vi "Sub Initialize.vi"(6 "Controller name":string, 8 "error in (no error)":errorcluster, 11 "Instrument Recorder in":refnum<class "DataSocket Client.lvclass">) -> (0 "error out":errorcluster, 2 "Initialize Result":refnum<class "Acquired Result.lvclass">, 3 "Instrument Recorder out":refnum<class "DataSocket Client.lvclass">)   [LabVIEW 2021, in "DataSocket Client.lvclass"]
uses:
  DataSocket Client.lvclass
  DataSocket Client.lvclass/DataSocket Client.ctl
  NHMFL_Core/Libraries/Instruments/Results/Start Stream Result/Start Stream Result.lvclass
  C:/GitHub/NHMFL_Core/Libraries/Instruments/Results/Acquired Result/Acquired Result.lvclass
  C:/GitHub/LabActor/Publish-Subscribe/Interfaces/Information/Information.lvclass
  C:/GitHub/NHMFL_Core/Libraries/Instruments/Results/Start Stream Result/Start Stream Result.lvclass
  NHMFL_Core/Libraries/Instruments/Results/Acquired Result/Acquired Result.lvclass
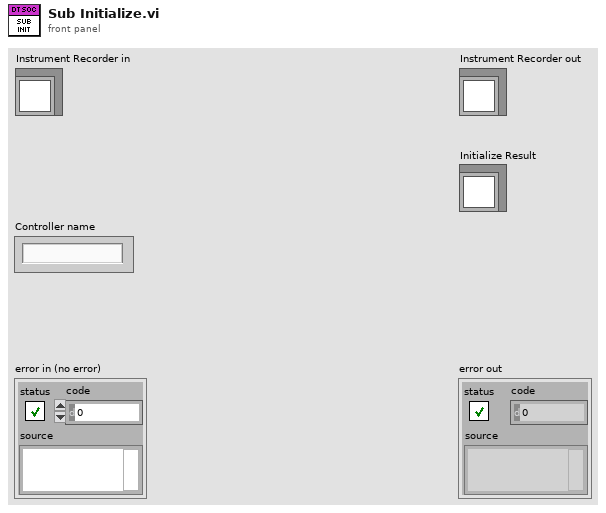
[diagram p1: front panel]
types:
  T1 = typedef "DataSocket Configuration.ctl" = cluster{"DataSocket  URLs":string[]}
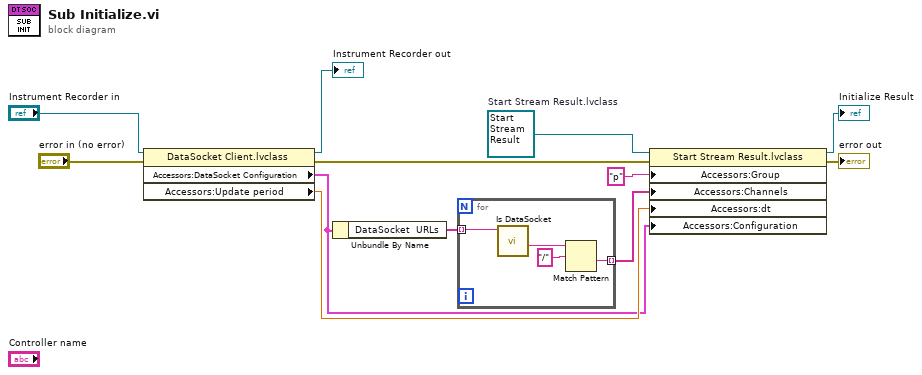
[diagram p0: block diagram]
diagram:
  w5 = refnum<class "Start Stream Result.lvclass"> refnum  # Start Stream Result.lvclass
  n1 = property class="DataSocket Client.lvclass"(reference="Instrument Recorder in", error in="error in (no error)") -> (reference out=→"Instrument Recorder out":refnum<class "DataSocket Client.lvclass">, error out=w4:errorcluster, "Accessors:DataSocket Configuration"=w6:T1, "Accessors:Update period"=w7:dbl)
  n2 = Unbundle By Name(w6) -> ("DataSocket  URLs"=w10:string[])
  n3 = for {
    tunnel: w10 -> [w16] mode=indexing
    tunnel: [w13] -> w8 mode=indexing
    n4 = call "Is DataSocket.vi"("String"=w16) -> ("After header"=w15:string)  [unwired: 9 in, 1 out]
    n5 = Match Pattern(string=w15, regular expression="/") -> (after substring=w13:string)  [unwired: 1 in, 3 out]
  }
  n6 = property class="Start Stream Result.lvclass"(reference=w5, error in=w4, "Accessors:Group"="p" ("Group"), "Accessors:Channels"=w8, "Accessors:dt"=w7, "Accessors:Configuration"=w6) -> (reference out=→"Initialize Result":refnum<class "Start Stream Result.lvclass">, error out=→"error out":errorcluster)
